vi "PRL UTIL Split Command.vi"(11 "Command":string) -> (2 "Parameters":string, 3 "Command Out":string)   [LabVIEW 2013, in "PMU Recorder Light.lvlib"]
doc: "Splits the command string into command and sub-command."
uses:
  PMU Recorder Light.lvlib
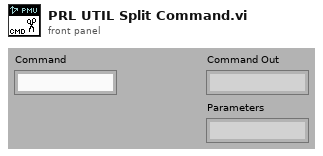
[diagram p1: front panel]
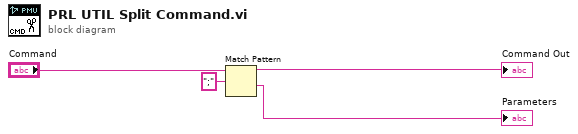
[diagram p0: block diagram]
diagram:
  n1 = Match Pattern(string="Command", regular expression=";") -> (before substring=→"Command Out":string, after substring=→"Parameters":string)  [unwired: 1 in, 2 out]
